vi "Write Response.vi"(0 "wait for ack (F)":bool, 1 "timeout in ms (-1)":i32=-1, 5 "element":T1, 7 "element valid? (T)":bool=TRUE, 9 "last element? (F)":bool, 11 "GUID":string, 12 "size (unlimited)":i32, 14 "abort (F)":bool) -> (3 "timed out?":bool, 4 "count":i32, 6 "channel":T2, 10 "id":u32, 15 "aborted?":bool)   [LabVIEW 2019, in "MessengerM.lvlib"]
doc: "Writes a response to a Messenger channel or signals the channel to abort. The endpoint waits if the channel is full. This endpoint is the same as the Write endpoint except that it has an <B>abort</B> input and an <B>aborted?</B> output. You can use the abort capability of the Messenger channel to close a channel abruptly, ignoring any data left in the channel buffer. You must use this endpoint together with the Read With Abort endpoint."
uses:
  <resource>/Channels/MessengerM/MessengerM.lvlib
  <resource>/Channels/MessengerM/EndpointOp.ctl
  <resource>/Channels/MessengerM/ParmsIn.ctl
  <resource>/Channels/MessengerM/))Channel.ctl
  <resource>/Channels/MessengerM/Element.ctl
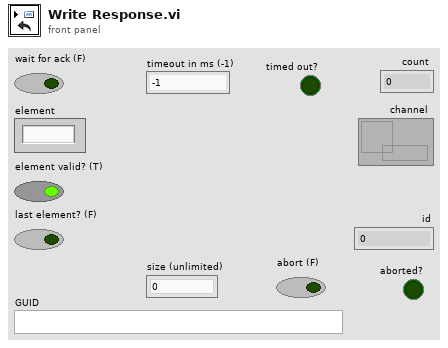
[diagram p1: front panel]
types:
  T1 = typedef "MessengerM.lvlib/Element.ctl" = string
  T2 = typedef "MessengerM.lvlib/))Channel.ctl" = refnum<queue>
  T3 = typedef "MessengerM.lvlib/ParmsIn.ctl" = cluster{"subchannel":i32, "size (0)":i32, "abort (F)":bool, "timeout":i32, "ack id (0)":u32, "last elt? (F)":bool, "valid? (T)":bool, "GUID":string}
  T4 = typedef "MessengerM.lvlib/EndpointOp.ctl" = enum16{"Write", "WriteAck", "WriteSync", "Read", "ReadAck"}
  T5 = typedef "MessengerM.lvlib/ParmsOut.ctl" = cluster{"count":i32, "aborted?":bool, "timedout?":bool, "id":u32, "last elt?":bool, "valid?":bool}
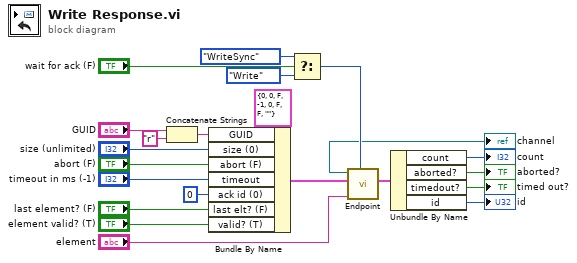
[diagram p0: block diagram]
diagram:
  n1 = Concatenate Strings("GUID", "r" ("string")) -> (w1:string)
  n2 = Bundle By Name(cluster=T3 {"subchannel"=0, "size (0)"=0, "abort (F)"=FALSE, "timeout"=-1, "ack id (0)"=0, "last elt? (F)"=FALSE, "valid? (T)"=FALSE, "GUID"=""} ("parms in"), "GUID"=w1, "size (0)"="size (unlimited)", "abort (F)"="abort (F)", "timeout"="timeout in ms (-1)", "ack id (0)"=u32 0, "last elt? (F)"="last element? (F)", "valid? (T)"="element valid? (T)") -> (w11:T3)
  n3 = Select(t=EndpointOp."WriteSync" ("endpointOp"), s="wait for ack (F)", f=EndpointOp."Write" ("endpointOp")) -> (s? t:f=w21:T4)
  n4 = call <resource>:"Endpoint.vi"("endpointOp"=w21, "element in"="element", "parms in"=w11, "channel in"="channel") -> ("parms out"=w10:T5)  [unwired: 6 in, 1 out]
  n5 = Unbundle By Name(w10) -> ("count"=→"count":i32, "aborted?"=→"aborted?":bool, "timedout?"=→"timed out?":bool, "id"=→"id":u32)
